vi "Write State.vi"(8 "error in (no error)":errorcluster, 10 "Current time":timestamp, 11 "Output Sequencer in":refnum<class "Output Sequencer.lvclass">) -> (0 "error out":errorcluster, 3 "Output Sequencer out":refnum<class "Output Sequencer.lvclass">)   [LabVIEW 2024, in "Output Sequencer.lvlib" / "Output Sequencer.lvclass"]
uses:
  Output Sequencer.lvclass
  C:/Program Files/National Instruments/LabVIEW 2024/vi.lib/FlexLogger/SDK/PluginSDK.lvlibp/PEFClasses/SDK/Plugin/Plugin.lvclass
  Output Sequencer.lvclass/Output Sequencer.ctl
  <vilib>/FlexLogger/SDK/PluginSDK.lvlibp/PEFClasses/SDK/Plugin/DataHelpers/Write 1D STR (NChan 1 Sample).vi
  <vilib>/FlexLogger/SDK/PluginSDK.lvlibp/PEFClasses/SDK/Plugin/Plugin.lvclass
  C:/Program Files/National Instruments/LabVIEW 2024/vi.lib/FlexLogger/SDK/PluginSDK.lvlibp/PEFClasses/SDK/Processing Element/Processing Element.lvclass
  C:/Dev/GitHub/ni/niflexlogger-plugins/PDK plugins/Output Sequencer/source/Output Sequencer/Output Sequencer.lvclass
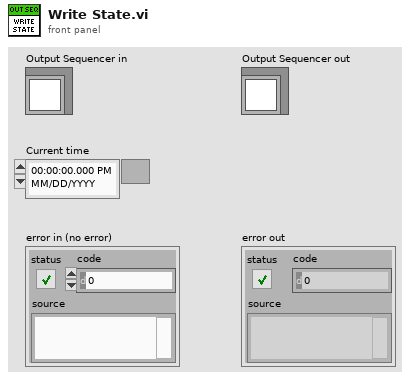
[diagram p1: front panel]
types:
  T1 = typedef "Output Sequencer.lvlib/Output Sequencer.lvclass/Sequencer State.ctl" = enum16{"Error", "Initialize", "Prepare channels", "Wait for test", "Wait for %.1f sec", "Wait for trigger", "Stop condition", "Wait for resume", "Running", "Paused", "No valid step", "Stopped"}
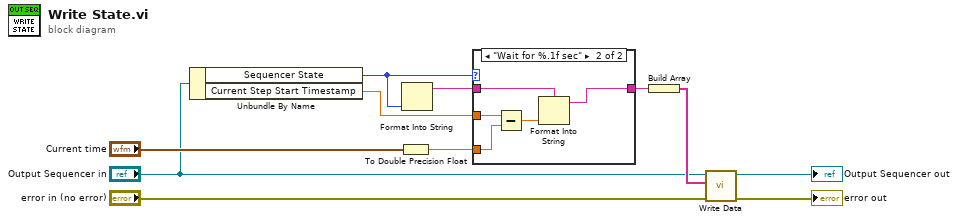
[diagram p0: block diagram]
diagram:
  n1 = Unbundle By Name("Output Sequencer in") -> ("Sequencer State"=w5:T1, "Current Step Start Timestamp"=w2:dbl)
  n2 = To Double Precision Float(number="Current time") -> (double precision float=w3:dbl)
  n3 = Format Into String(w5) -> (resulting string=w8:string)  [unwired: 3 in, 1 out]
  n4 = case shown="\"Wait for %.1f sec\"" w5 {
    tunnel: w8 -> [w12 w17]
    tunnel: w2 -> [_ w15]
    tunnel: [w12 w16] -> w7
    tunnel: w3 -> [_ w14]
    frame Default {
    }
    frame "Wait for %.1f sec" {
      n5 = Subtract(x=w15, y=w14) -> (x-y=w13:dbl)
      n6 = Format Into String(format string=w17, w13) -> (resulting string=w16:string)  [unwired: 2 in, 1 out]
    }
  }
  n7 = Build Array(w7) -> (w6:string[])
  n8 = call-poly <vilib>:"Write Data.vi"("error in (no error)"="error in (no error)", "Data"=w6, "Plugin in"="Output Sequencer in") -> ("error out"=→"error out":errorcluster, "Plugin out"=→"Output Sequencer out":refnum<class "Output Sequencer.lvclass">)  [unwired: 7 in]
